vi "Create UA Server Tree.vi"(8 "Error In":errorcluster, 9 "Display Name":string, 11 "Server Endpoint URL (Root folder)":string) -> (0 "Error Out":errorcluster, 3 "UA Server Tree":refnum<class "UA Server.lvclass">)   [LabVIEW 2017, in "opcua.lvlib" / "Browser Core.lvlib" / "UA Server.lvclass"]
doc: "Create OPC UA tree structure with root id. When the tree is created, a client connection to the OPC UA server will also be established."
uses:
  UA Server.lvclass
  UA Server.lvclass/UA Server.ctl
  Base Tree/Base Tree.lvclass
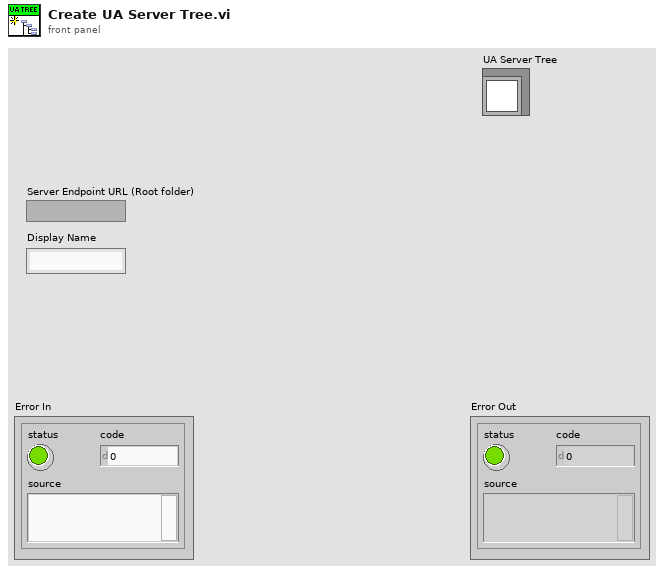
[diagram p1: front panel]
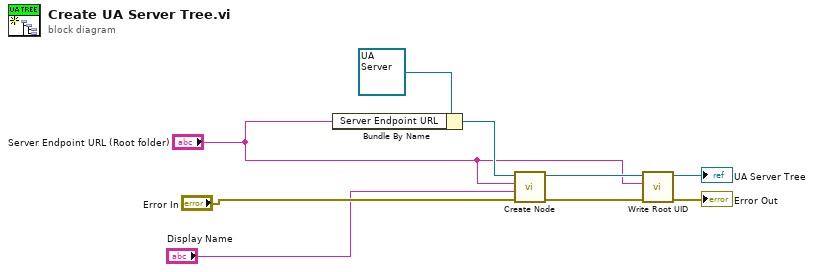
[diagram p0: block diagram]
diagram:
  n1 = Bundle By Name(cluster=refnum<class "UA Server.lvclass"> refnum ("UA Server Tree"), "Server Endpoint URL"="Server Endpoint URL (Root folder)") -> (w8:refnum<class "UA Server.lvclass">)
  n2 = call "Create Node.vi"("error in (no error)"="Error In", "Display Name"="Display Name", "UID"="Server Endpoint URL (Root folder)", "Base Tree in"=w8) -> ("error out"=w7:errorcluster, "Base Tree out"=w6:refnum<class "UA Server.lvclass">)  [unwired: 6 in]
  n3 = call "Write Root UID.vi"("error in (no error)"=w7, "Root UID"="Server Endpoint URL (Root folder)", "Base Tree in"=w6) -> ("error out"=→"Error Out":errorcluster, "Base Tree out"=→"UA Server Tree":refnum<class "UA Server.lvclass">)  [unwired: 7 in]
